vi "DHE_GetModRef.vi"() -> (7 "DHE_ModRef":refnum<vi>)   [LabVIEW 2016]
uses:
  DHE_GBLDriverVariables.vi
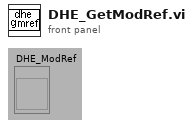
[diagram p1: front panel]
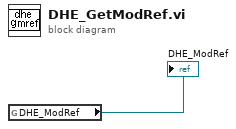
[diagram p0: block diagram]
diagram:
  n1 = global read "DHE_GBLDriverVariables.vi" "DHE_ModRef"() -> (→"DHE_ModRef":refnum<vi>)
